vi "VI Methods - Row 1.vi"(7 "Format Options":T1={"Background"={"Public Scope"={"Option"=FALSE, "Color"=0, "Operator"=FALSE}, "Protected Scope"={"Option"=FALSE, "Color"=0, "Operator"=FALSE}, "Community Scope"={"Option"=FALSE, "Color"=0, "Operator"=FALSE}, "Private Scope"={"Option"=FALSE, "Color"=0, "Operator"=FALSE}, "Unknown Scope"={"Option"=FALSE, "Color"=0, "Operator"=FALSE}, "Auto Error Handling"={"Option"=FALSE, "Color"=0, "Operator"=FALSE}, "Inline"={"Option"=FALSE, "Color"=0, "Operator"=FALSE}, "Separate CC"={"Option"=FALSE, "Color"=0, "Operator"=FALSE}, "Execution Priority Normal"={"Option"=FALSE, "Color"=0, "Operator"=FALSE}, "Reentrancy Non-RE"={"Option"=FALSE, "Color"=0, "Operator"=FALSE}}, "Bookmark Options"={"Bookmarks as New Line in VI Descriptions"=TRUE, "Unique Bookmark Tags Only"=TRUE, "Include Tag and Text"=TRUE}}, 8 "Error in":errorcluster caption="Error in (no error)", 11 "VI Info":T4 caption="cluster") -> (0 "Error out":errorcluster, 1 "Column Headers":string[](array[string])=["Name", "Reentrant", "Inline", "Auto Error", "Compiled"], 3 "Table Row Text":string)   [LabVIEW 2023, in "VIDoc Printer - Confluence.lvlib" / "VIDoc Printer - Confluence.lvclass"]
uses:
  VIDoc Printer - Confluence.lvclass
  Parsing/TypeDefs/Method Spec Cluster.ctl
  Parsing/TypeDefs/VI Type Extended Enum.ctl
  <vilib>/picture/picture.llb/imagedata.ctl
  Parsing/TypeDefs/Class Dispatch Type Enum.ctl
  Parsing/TypeDefs/Controls Info Cluster.ctl
  <vilib>/Utility/miscctls.llb/LVKeyTypeDef.ctl
  <vilib>/Utility/miscctls.llb/LVPointTypeDef.ctl
  Parsing/SubVIs/Structure Reporter/Tree Cluster.ctl
  Settings/Printer Settings/Formatting Options.ctl
  Settings/Printer Settings/Background Formatting Cluster.ctl
  Settings/Printer Settings/Bookmark Options.ctl
  VIDoc Printer - Confluence.lvclass/VIDoc Printer - Confluence.ctl
  Confluence Formatting/Confluence Formatting.lvlib
  Printer/VIDoc Printer.lvclass
  Parsing/VIDoc Parsing.lvlib
  Settings/Printer Settings/Printer Settings.lvclass
  Parsing/SubVIs/Structure Reporter/Structure Reporter.lvlib
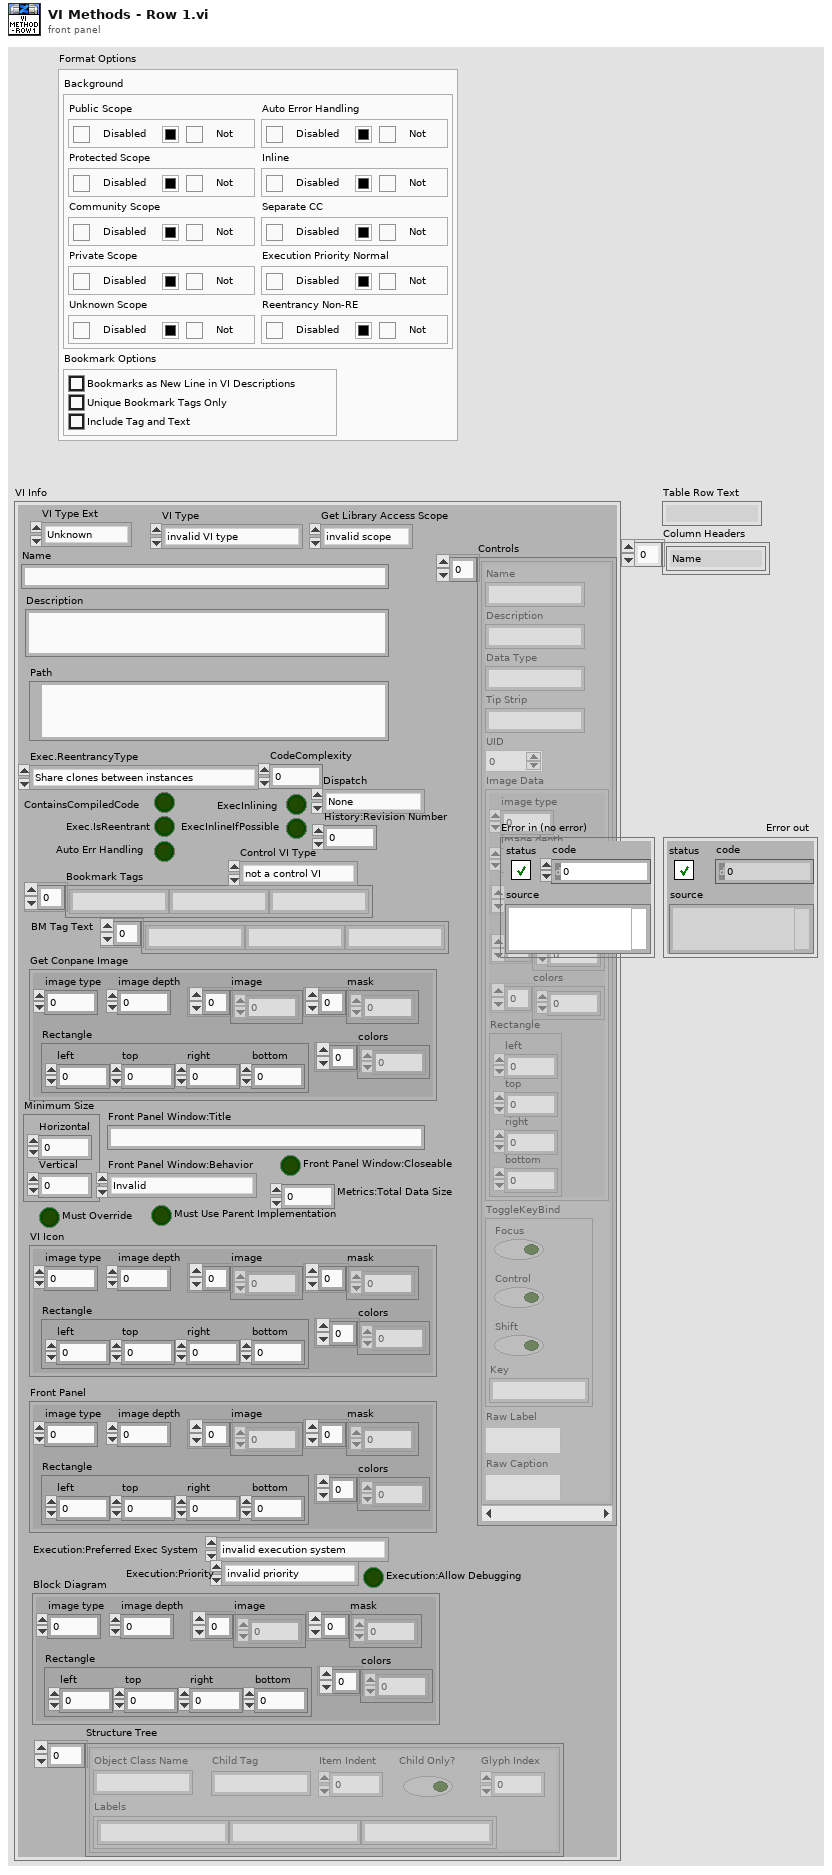
[diagram p1: front panel]
types:
  T1 = typedef "VIDoc Printer.lvlib/Printer Settings.lvclass/Formatting Options.ctl" = cluster{"Background":cluster{"Public Scope":T2, "Protected Scope":T2, "Community Scope":T2, "Private Scope":T2, "Unknown Scope":T2, "Auto Error Handling":T2, "Inline":T2, "Separate CC":T2, "Execution Priority Normal":T2, "Reentrancy Non-RE":T2}, "Bookmark Options":T3}
  T2 = typedef "VIDoc Printer.lvlib/Printer Settings.lvclass/Background Formatting Cluster.ctl" = cluster{"Option":bool, "Color":u32, "Operator":bool}
  T3 = typedef "VIDoc Printer.lvlib/Printer Settings.lvclass/Bookmark Options.ctl" = cluster{"Bookmarks as New Line in VI Descriptions":bool, "Unique Bookmark Tags Only":bool, "Include Tag and Text":bool}
  T4 = typedef "VIDoc Parsing.lvlib/Method Spec Cluster.ctl" = cluster{"VI Type Ext":T5, "Name":string, "Path":path, "Get Conpane Image":T6, "Description":string, "Get Library Access Scope":enum32{"invalid scope", "public", "private", "protected", "community"}, "Dispatch":T7, "ContainsCompiledCode":bool, "Exec.IsReentrant":bool, "Exec.ReentrancyType":enum16{"Share clones between instances", "Preallocate clone for each instance"}, "ExecInlining":bool, "ExecInlineIfPossible":bool, "Auto Err Handling":bool, "CodeComplexity":sgl, "Bookmark Tags":string[], "Control VI Type":enum32{"not a control VI", "control", "typedef", "strict typedef"}, "Controls":T8[], "VI Type":enum32{"invalid VI type", "Standard VI", "Control VI", "Global VI", "Polymorphic VI", "Configuration VI", "SubSystem", "Facade VI", "Method VI", "Statechart Diagram VI"}, "Minimum Size":T10, "Front Panel Window:Title":string, "Front Panel Window:Behavior":enum32{"Invalid", "Default", "Floating", "Floating/Auto-Hide", "Modal"}, "Front Panel Window:Closeable":bool, "Must Override":bool, "Must Use Parent Implementation":bool, "VI Icon":T6, "Front Panel":T6, "History:Revision Number":u32, "Metrics:Total Data Size":u32, "Execution:Allow Debugging":bool, "Execution:Preferred Exec System":enum32{"invalid execution system", "user interface", "standard", "instrument i/o", "data acquisition", "other 1", "other 2", "same as caller"}, "Execution:Priority":enum32{"invalid priority", "background priority", "normal priority", "above normal priority", "high priority", "time critical priority", "subroutine"}, "BM Tag Text":string[], "Block Diagram":T6, "Structure Tree":T11[]}
  T5 = typedef "VIDoc Parsing.lvlib/VI Type Extended Enum.ctl" = enum16{"Unknown", "Class Method", "Class Accessor Get", "Class Accessor Set", "Class Control", "Library Method", "Library Control", "VI", "Control"}
  T6 = typedef "imagedata.ctl" = cluster{"image type":i32, "image depth":i32, "image":u8[], "mask":u8[], "colors":u32[], "Rectangle":cluster{"left":i16, "top":i16, "right":i16, "bottom":i16}}
  T7 = typedef "VIDoc Parsing.lvlib/Class Dispatch Type Enum.ctl" = enum16{"None", "Static", "Dynamic"}
  T8 = typedef "VIDoc Parsing.lvlib/Controls Info Cluster.ctl" = cluster{"Name":string, "Description":string, "Data Type":string, "Tip Strip":string, "UID":i32, "Image Data":T6, "ToggleKeyBind":T9, "Raw Label":string, "Raw Caption":string}
  T9 = typedef "LVKeyTypeDef.ctl" = cluster{"Focus":bool, "Control":bool, "Shift":bool, "Key":string}
  T10 = typedef "LVPointTypeDef.ctl" = cluster{"Horizontal":i16, "Vertical":i16}
  T11 = typedef "VIDoc Parsing.lvlib/Structure Reporter.lvlib/Tree Cluster.ctl" = cluster{"Object Class Name":string, "Labels":string[], "Child Tag":string, "Item Indent":i32, "Child Only?":bool, "Glyph Index":i32}
  T12 = enum16{"Share clones between instances", "Preallocate clone for each instance"}
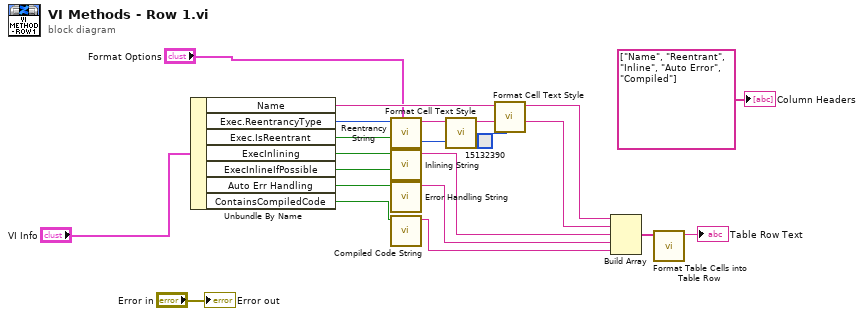
[diagram p0: block diagram]
diagram:
  n1 = Unbundle By Name("VI Info") -> ("Name"=w6:string, "Exec.ReentrancyType"=w11:T12, "Exec.IsReentrant"=w12:bool, "ExecInlining"=w14:bool, "ExecInlineIfPossible"=w15:bool, "Auto Err Handling"=w18:bool, "ContainsCompiledCode"=w20:bool)
  n2 = call "Reentrancy String.vi"("Format Options"="Format Options", "Exec.IsReentrant"=w12, "Exec.ReentrancyType"=w11) -> ("Cell Color"=w2:u32, "Reentrancy"=w13:string)  [unwired: 7 in]
  n3 = call "Inlining String.vi"("ExecInlineIfPossible"=w15, "ExecInlining"=w14) -> ("Inline Text"=w17:string)  [unwired: 9 in]
  n4 = call "Error Handling String.vi"("Auto Err Handling"=w18) -> ("Error Handling String"=w19:string)  [unwired: 10 in]
  n5 = call "Compiled Code String.vi"("ContainsCompiledCode"=w20) -> ("Compiled Code String"=w21:string)  [unwired: 10 in]
  n6 = call "Format Cell Text Style.vi"("BG Color (Unchanged)"=w2, "String"=w13) -> ("Formatted Text"=w16:string)  [unwired: 8 in, 1 out]
  n7 = call "Format Cell Text Style.vi"("BG Color (Unchanged)"=u32 15132390, "String"=w6) -> ("Formatted Text"=w7:string)  [unwired: 8 in, 1 out]
  n8 = Build Array(w7, w16, w17, w19, w21) -> (w8:string[])
  n9 = call "Format Table Cells into Table Row.vi"("Table Cells"=w8) -> ("Table Row Text"=→"Table Row Text":string)  [unwired: 10 in]
  "Error out" <- "Error in"
  "Column Headers" <- string[] ["Name", "Reentrant", "Inline", "Auto Error", "Compiled"]
